vi "PointOverlay-Dual channel.vi"(8 "Coordinates":cluster{"X":i32, "Y":i32}, 9 "Count":i32, 10 "Image2":T1, 11 "Image1":T1) -> (2 "Image2 Out":T1, 3 "Image1 Out":T1)   [LabVIEW 2017]
uses:
  <vilib>/vision/Image Controls.llb/IMAQ Image.ctl
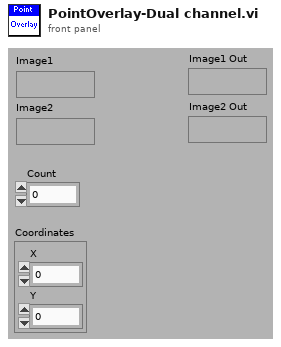
[diagram p1: front panel]
types:
  T1 = typedef "IMAQ Image.ctl" = refnum<image>
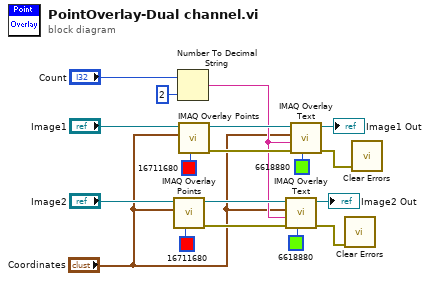
[diagram p0: block diagram]
diagram:
  n1 = call "IMAQ Overlay Points"("Color"=u32 16711680, "Point"="Coordinates", "Image"="Image2") -> ("error out"=w15:errorcluster, "Image Out"=w14:T1)  [unwired: 7 in]
  n2 = Number To Decimal String(number="Count", width (-)=i16 2) -> (decimal integer string=w9:string)
  n3 = call "IMAQ Overlay Points"("Color"=u32 16711680, "Point"="Coordinates", "Image"="Image1") -> ("error out"=w12:errorcluster, "Image Out"=w13:T1)  [unwired: 7 in]
  n4 = call "IMAQ Overlay Text"("Text Color (black)"=u32 6618880, "error in (no error)"=w15, "String"=w9, "Origin"="Coordinates", "Image"=w14) -> ("error out"=w1:errorcluster, "Image Out"=→"Image2 Out":T1)  [unwired: 5 in]
  n5 = call "IMAQ Overlay Text"("Text Color (black)"=u32 6618880, "error in (no error)"=w12, "String"=w9, "Origin"="Coordinates", "Image"=w13) -> ("error out"=w2:errorcluster, "Image Out"=→"Image1 Out":T1)  [unwired: 5 in]
  n6 = call <vilib>:"Clear Errors.vi"("error in (no error)"=w1) -> ()  [unwired: 5 in, 2 out]
  n7 = call <vilib>:"Clear Errors.vi"("error in (no error)"=w2) -> ()  [unwired: 5 in, 2 out]
